vi "encodeFloat32.vi"(3 "Float32":sgl) -> (1 "MessagePack":u8[](array[numeric]) format="%.0x")   [LabVIEW 2015, in "MsgPack.lvlib"]
uses:
  MsgPack.lvlib
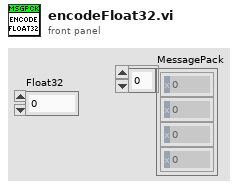
[diagram p1: front panel]
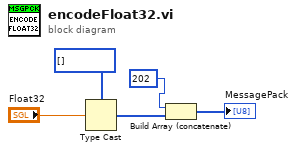
[diagram p0: block diagram]
diagram:
  n1 = Type Cast(type=u8[] [], x="Float32") -> (*(type *) &x=w3:u8[])
  n2 = Build Array (concatenate)(u8 202, w3) -> (→"MessagePack":u8[])
